vi "XNET Database Remove Alias.vi"(5 "alias":string, 11 "error in (no error)":errorcluster) -> (15 "error out":errorcluster)   [LabVIEW 2018]
doc: "Removes a database alias from the system."
uses:
  nixlvapi.dll
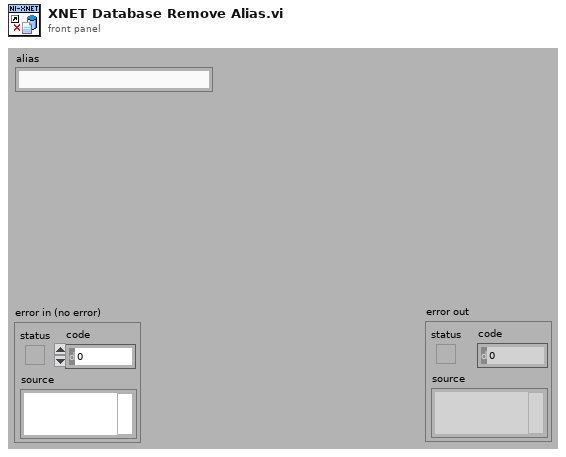
[diagram p1: front panel]
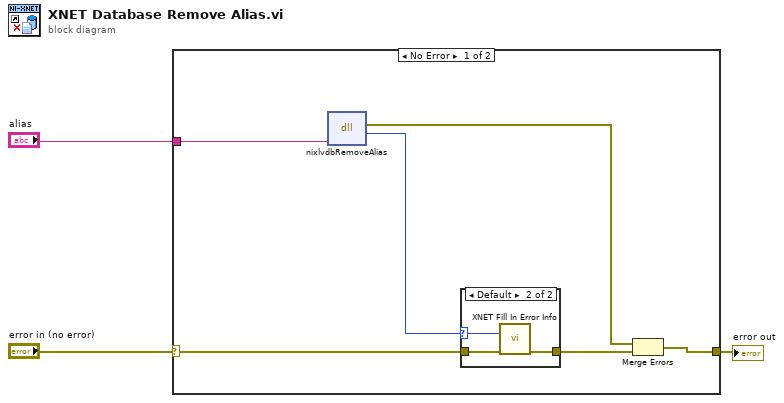
[diagram p0: block diagram]
diagram:
  n1 = case shown="No Error" "error in (no error)" {
    selector: "error in (no error)" -> [w8 w14]
    tunnel: "alias" -> [w6 _]
    tunnel: [w5 w14] -> w3
    frame No Error {
      n2 = dll-call lib="nixlvapi.*" fn="nixlvdbRemoveAlias" ("nilvxaiu.dll:lvxenDatabaseDeleteObject")("DatabaseAlias"=w6) -> (error out=w4:errorcluster, "return type"=w7:i32)  [unwired: 4 in, 1 out]
      n3 = case shown="Default" w7 {
        selector: w7 -> [_ w11]
        tunnel: w8 -> [w10 w12]
        tunnel: [w10 w13] -> w9
        frame 0 {
        }
        frame Default {
          n4 = call "XNET Fill In Error Info.vi"("status code"=w11, "error in"=w12) -> ("error out"=w13:errorcluster)  [unwired: 13 out]
        }
      }
      n5 = Merge Errors(w4, w9) -> (w5:errorcluster)
    }
    frame Error {
    }
  }
  "error out" <- w3
